vi "ToFeedForwardData.vi"(9 "values Q":dbl[](array[numeric]), 10 "values I":dbl[](array[numeric]), 11 "Memory block":T1) -> (3 "Data":u64[](array[numeric]))   [LabVIEW 2013]
uses:
  controls/Memory block.ctl
  <vilib>/rvi/FXPMathLib/FxpInterpret/XNode/nifxpmath_Interpret.xnode
  <userlib>/_OpenG.lib/numeric/numeric.llb/Random Number Within Range - DBL__ogtk.vi
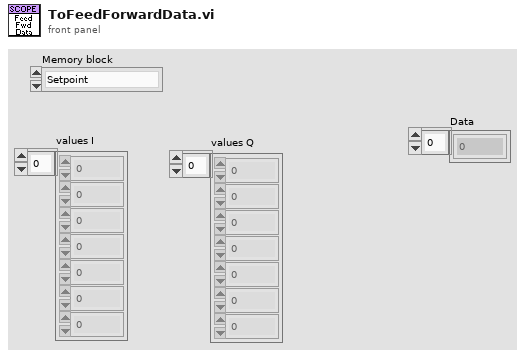
[diagram p1: front panel]
types:
  T1 = typedef "Memory block.ctl" = enum16{"Setpoint", "Beam"}
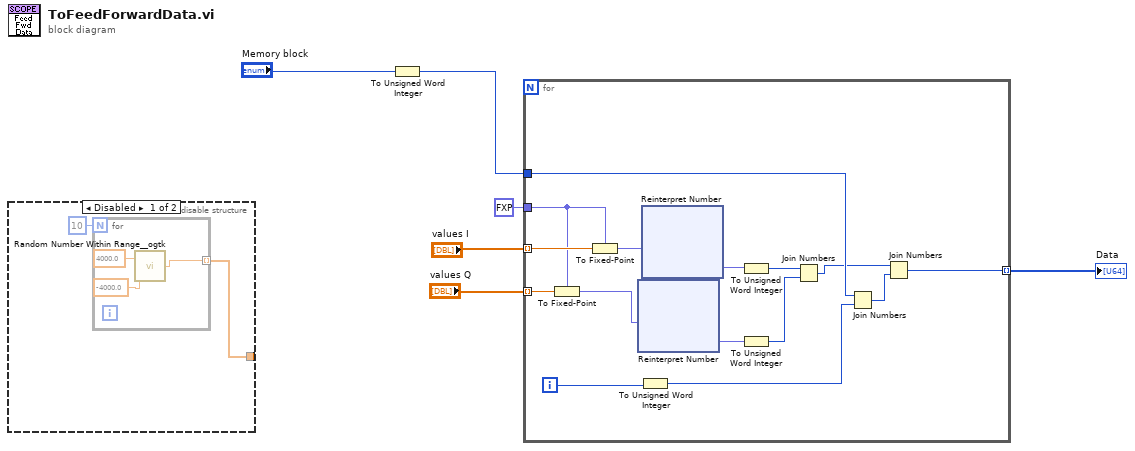
[diagram p0: block diagram]
diagram:
  n1 = disable-structure shown="Disabled" {
    disable-tunnel: [w7 _] -> _
    frame Disabled {
      n2 = for {
        N: 10 -> [_]
        tunnel: [w9] -> w7 mode=indexing
        n3 = call-poly <userlib>:"Random Number Within Range__ogtk.vi"("High"=4000.0, "Low"=-4000.0 ("High")) -> ("Random Number"=w9:dbl)  [unwired: 3 in]
      }
    }
    frame Enabled {
    }
  }
  n4 = To Unsigned Word Integer(number="Memory block") -> (unsigned 16bit integer=w5:u16)
  n5 = for {
    tunnel: fxp<+/-,16,14> 0.0 ("fixed-point type") -> [w21]
    tunnel: w5 -> [w25]
    tunnel: [w24] -> w1 mode=indexing
    tunnel: "values I" -> [w23] mode=indexing
    tunnel: "values Q" -> [w22] mode=indexing
    i -> [w14]
    n6 = To Fixed-Point(fixed-point type=w21, number=w22) -> (fixed-point=w20:fxp<+/-,16,14>)
    n7 = To Fixed-Point(fixed-point type=w21, number=w23) -> (fixed-point=w26:fxp<+/-,16,14>)
    n8 = xnode "Reinterpret Number"("x"=w20) -> ("y"=w19:fxp<+,16,16>)
    n9 = To Unsigned Word Integer(number=w14) -> (unsigned 16bit integer=w13:u16)
    n10 = xnode "Reinterpret Number"("x"=w26) -> ("y"=w18:fxp<+,16,16>)
    n11 = To Unsigned Word Integer(number=w18) -> (unsigned 16bit integer=w17:u16)
    n12 = To Unsigned Word Integer(number=w19) -> (unsigned 16bit integer=w12:u16)
    n13 = Join Numbers(hi=w17, lo=w12) -> ((hi.lo)=w16:u32)
    n14 = Join Numbers(hi=w25, lo=w13) -> ((hi.lo)=w15:u32)
    n15 = Join Numbers(hi=w16, lo=w15) -> ((hi.lo)=w24:u64)
  }
  "Data" <- w1
